vi "PhysionetReaderPresentation.vi"() -> ()   [LabVIEW 2012]
panel:
  in  "numer sygnału":i32
  out "Waveform Graph":waveform(dbl)(graph)
  in  "Combo Box":string(combo)
  in  "stop":bool
  in  "Folder Path":path
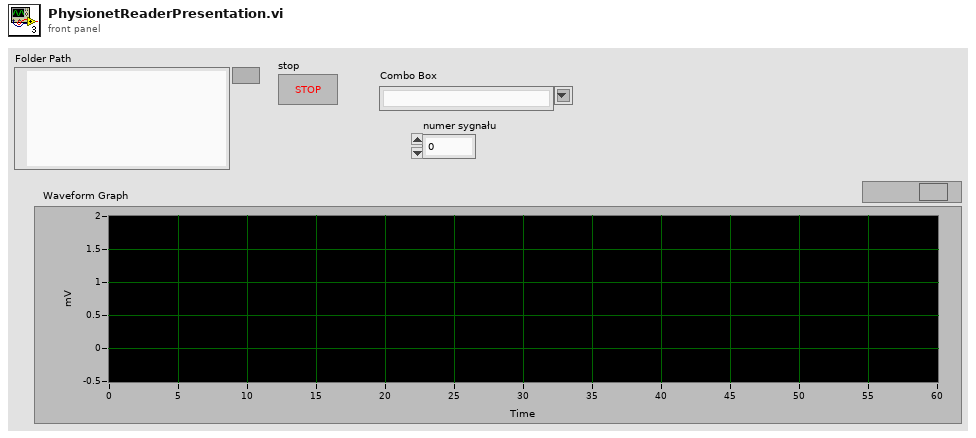
[diagram p1: front panel]
types:
  T1 = typedef "#typedef_SignalSpecInfo.ctl" = cluster{"file name":string, "format":i32, "samples per frame":i32, "skew":i32, "byte offset":i32, "ADC gain":dbl, "baseline (ADC units)":i32, "units":string, "ADC resolution":i16, "ADC zero":i16, "initial value":i16, "checksum":i16, "block size":i32, "description":string}
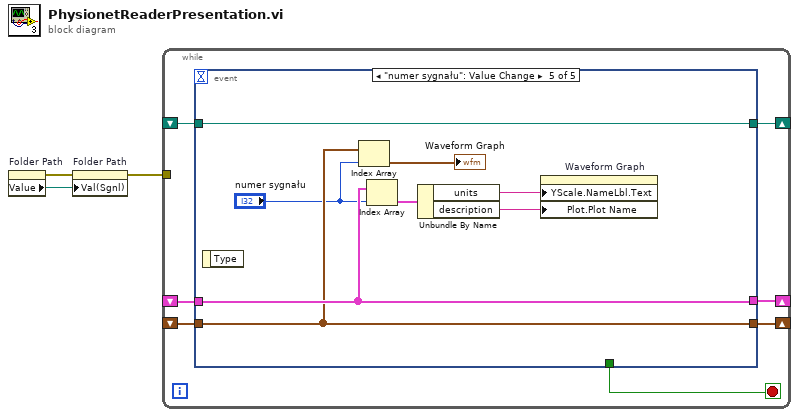
[diagram p0: block diagram]
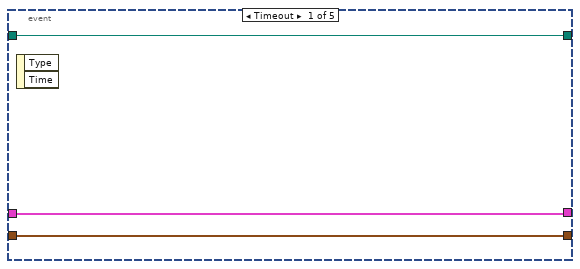
[diagram p2: hidden frame]
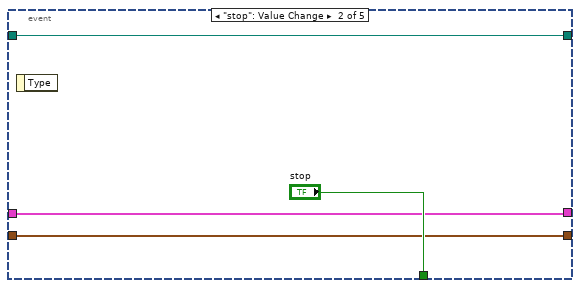
[diagram p3: hidden frame]
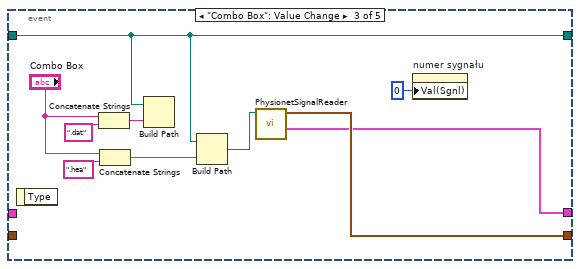
[diagram p4: hidden frame]
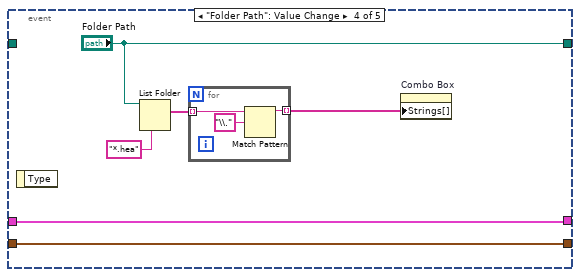
[diagram p5: hidden frame]
diagram:
  n1 = property on="Folder Path" class="Path"() -> (error out=w1:errorcluster, "Value"=w2:path)  [unwired: 2 in, 1 out]
  n2 = property on="Folder Path" class="Path"(error in=w1, "Val(Sgnl)"=w2) -> (error out=w3:errorcluster)  [unwired: 1 in, 1 out]
  n3 = while {
    shift-right: [w9] -> _
    shift-left: _ -> [w8]
    shift-right: [w7] -> _
    shift-left: _ -> [w6]
    shift-right: [w5] -> _
    shift-left: _ -> [w4]
    tunnel: w3 -> [_]
    stop <- w10 stop-if-true
    n4 = event shown="[4] \"numer sygnału\": Value Change" {
      selector: _ -> [_ _ _ _ _]
      dyn-events: _ -> [_ _ _ _ _]
      timeout: _ -> [_ _ _ _ _]
      tunnel: [_ "stop" _ _ _] -> w10
      tunnel: [w13 w16 w18 "Folder Path" w37] -> w9
      tunnel: w8 -> [w13 w16 w18 _ w37]
      tunnel: [w12 w15 w22 w29 w41] -> w7
      tunnel: w6 -> [w12 w15 _ w29 w41]
      tunnel: [w11 w14 w21 w28 w43] -> w5
      tunnel: w4 -> [w11 w14 _ w28 w43]
      event Timeout {
        n5 = event-data() -> ()  [unwired: 1 in, 2 out]
      }
      event "stop": Value Change {
        n6 = event-data() -> ()  [unwired: 1 in, 1 out]
      }
      event "Combo Box": Value Change {
        n7 = event-data() -> ()  [unwired: 1 in, 1 out]
        n8 = Concatenate Strings("Combo Box", ".dat" ("string")) -> (w25:string)
        n9 = Concatenate Strings("Combo Box", ".hea" ("string")) -> (w24:string)
        n10 = Build Path(base path=w18, name or relative path=w25) -> ()  [unwired: 1 out]
        n11 = Build Path(base path=w18, name or relative path=w24) -> (appended path=w19:path)
        n12 = call "PhysionetSignalReader.vi"("Header file path"=w19) -> ("Signals Specs Info"=w21:T1[], "Signals(physical units)"=w22:waveform(dbl)[])  [unwired: 6 in, 3 out]
        n13 = property on="numer sygnału" class="DigNum (strict)"("Val(Sgnl)"=0 ("Value (Signaling)")) -> ()  [unwired: 2 in, 2 out]
      }
      event "Folder Path": Value Change {
        n14 = event-data() -> ()  [unwired: 1 in, 1 out]
        n15 = List Folder(path="Folder Path", pattern="*.hea") -> (filenames=w32:string[])  [unwired: 2 in, 3 out]
        n16 = for {
          tunnel: w32 -> [w36] mode=indexing
          tunnel: [w34] -> w33 mode=indexing
          n17 = Match Pattern(string=w36, regular expression="\\.") -> (before substring=w34:string)  [unwired: 1 in, 3 out]
        }
        n18 = property on="Combo Box" class="CmbBox"("Strings[]"=w33) -> ()  [unwired: 2 in, 2 out]
      }
      event "numer sygnału": Value Change {
        n19 = event-data() -> ()  [unwired: 1 in, 1 out]
        n20 = Index Array(array=w41, index="numer sygnału") -> (element=→"Waveform Graph":waveform(dbl))
        n21 = Index Array(array=w43, index="numer sygnału") -> (element=w42:T1)
        n22 = Unbundle By Name(w42) -> ("units"=w38:string, "description"=w44:string)
        n23 = property on="Waveform Graph" class="WFGraph (strict)"("YScale.NameLbl.Text"=w38, "Plot.Plot Name"=w44) -> ()  [unwired: 2 in, 2 out]
      }
    }
  }
